vi "SV Convert to Data Object.vi"   [LabVIEW 2017, in "Data.lvclass"]
doc: "Use this polymorphic VI to convert spectra to a class data type that you can view on the Spectrum with Cursors XControl. You must manually select the polymorphic instance to use."
uses:
  <vilib>/addons/_NISVFA/_Shared subVIs/Data Objects/Data/Data.lvclass
  <vilib>/addons/_NISVFA/_Shared subVIs/Data Objects/Y (DBL)/Y (1 Ch).lvclass
  <vilib>/addons/_NISVFA/_Shared subVIs/Data Objects/Y (DBL)/Y (N Ch).lvclass
  <vilib>/addons/_NISVFA/_Shared subVIs/Data Objects/Y (Complex) (DBL)/Y (Complex) (1 Ch).lvclass
  <vilib>/addons/_NISVFA/_Shared subVIs/Data Objects/Y (Complex) (DBL)/Y (Complex) (N Ch).lvclass
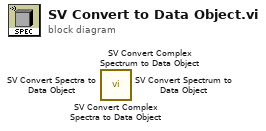
[diagram p0: block diagram]
diagram:
  n1 = call <vilib>:"SV Convert Complex Spectra to Data Object.vi"() -> ()  [unwired: 18 in, 2 out]
  n2 = call <vilib>:"SV Convert Complex Spectrum to Data Object.vi"() -> ()  [unwired: 18 in, 2 out]
  n3 = call <vilib>:"SV Convert Spectra to Data Object.vi"() -> ()  [unwired: 18 in, 2 out]
  n4 = call <vilib>:"SV Convert Spectrum to Data Object.vi"() -> ()  [unwired: 18 in, 2 out]
